vi "生成MES数据串.vi"(7 "测试结果":string, 8 "error in (no error)":errorcluster caption="错误输入（无错误）", 9 "操作状态":T1(ring), 10 "MES配置":T2={"接口地址："="http://192.168.100.120:50000/manufacturing/IntegrationServlet?InterType=XML&message=", "SITE（站点）   "="A155", "PWD（口令）"="LTF", "RESOURCE（资源）"="123456", "OPERATION（工序）"="B03-DZ-ZSCX-01", "USER（用户）"="DZ-ZSCX", "QTY"="LTF", "ACTIVITY"="1", "NC_CODE（NG代码）"="XML", "启用MES"=FALSE}, 11 "ID(SN)":string="A155001") -> (0 "error out":errorcluster caption="错误输出", 2 "Data(OUT)":string="http://192.168.100.120:50000/manufacturing/IntegrationServlet?InterType=XML&message=<PRODUCTION_REQUEST><USER><SITE>A155</SITE><NAME>LTF</NAME><PWD>123456</PWD></USER></PRODUCTION_REQUEST>")   [LabVIEW 2011]
doc: "Power by Antenna~"
panel:
  in  "字符串":string
  out "连接的字符串":string
  out "Data(OUT) 2":string="http://192.168.100.120:50000/manufacturing/IntegrationServlet?InterType=XML&message=<PRODUCTION_REQUEST><USER><SITE>A155</SITE><NAME>LTF</NAME><PWD>123456</PWD></USER></PRODUCTION_REQUEST>"
  # "Name和User有什么\n区别呢？？"
  # "QTY\n默认值为1"
  # "注意中划线和下划线；\n注意大小写；\n注意全角字符和半角字符"
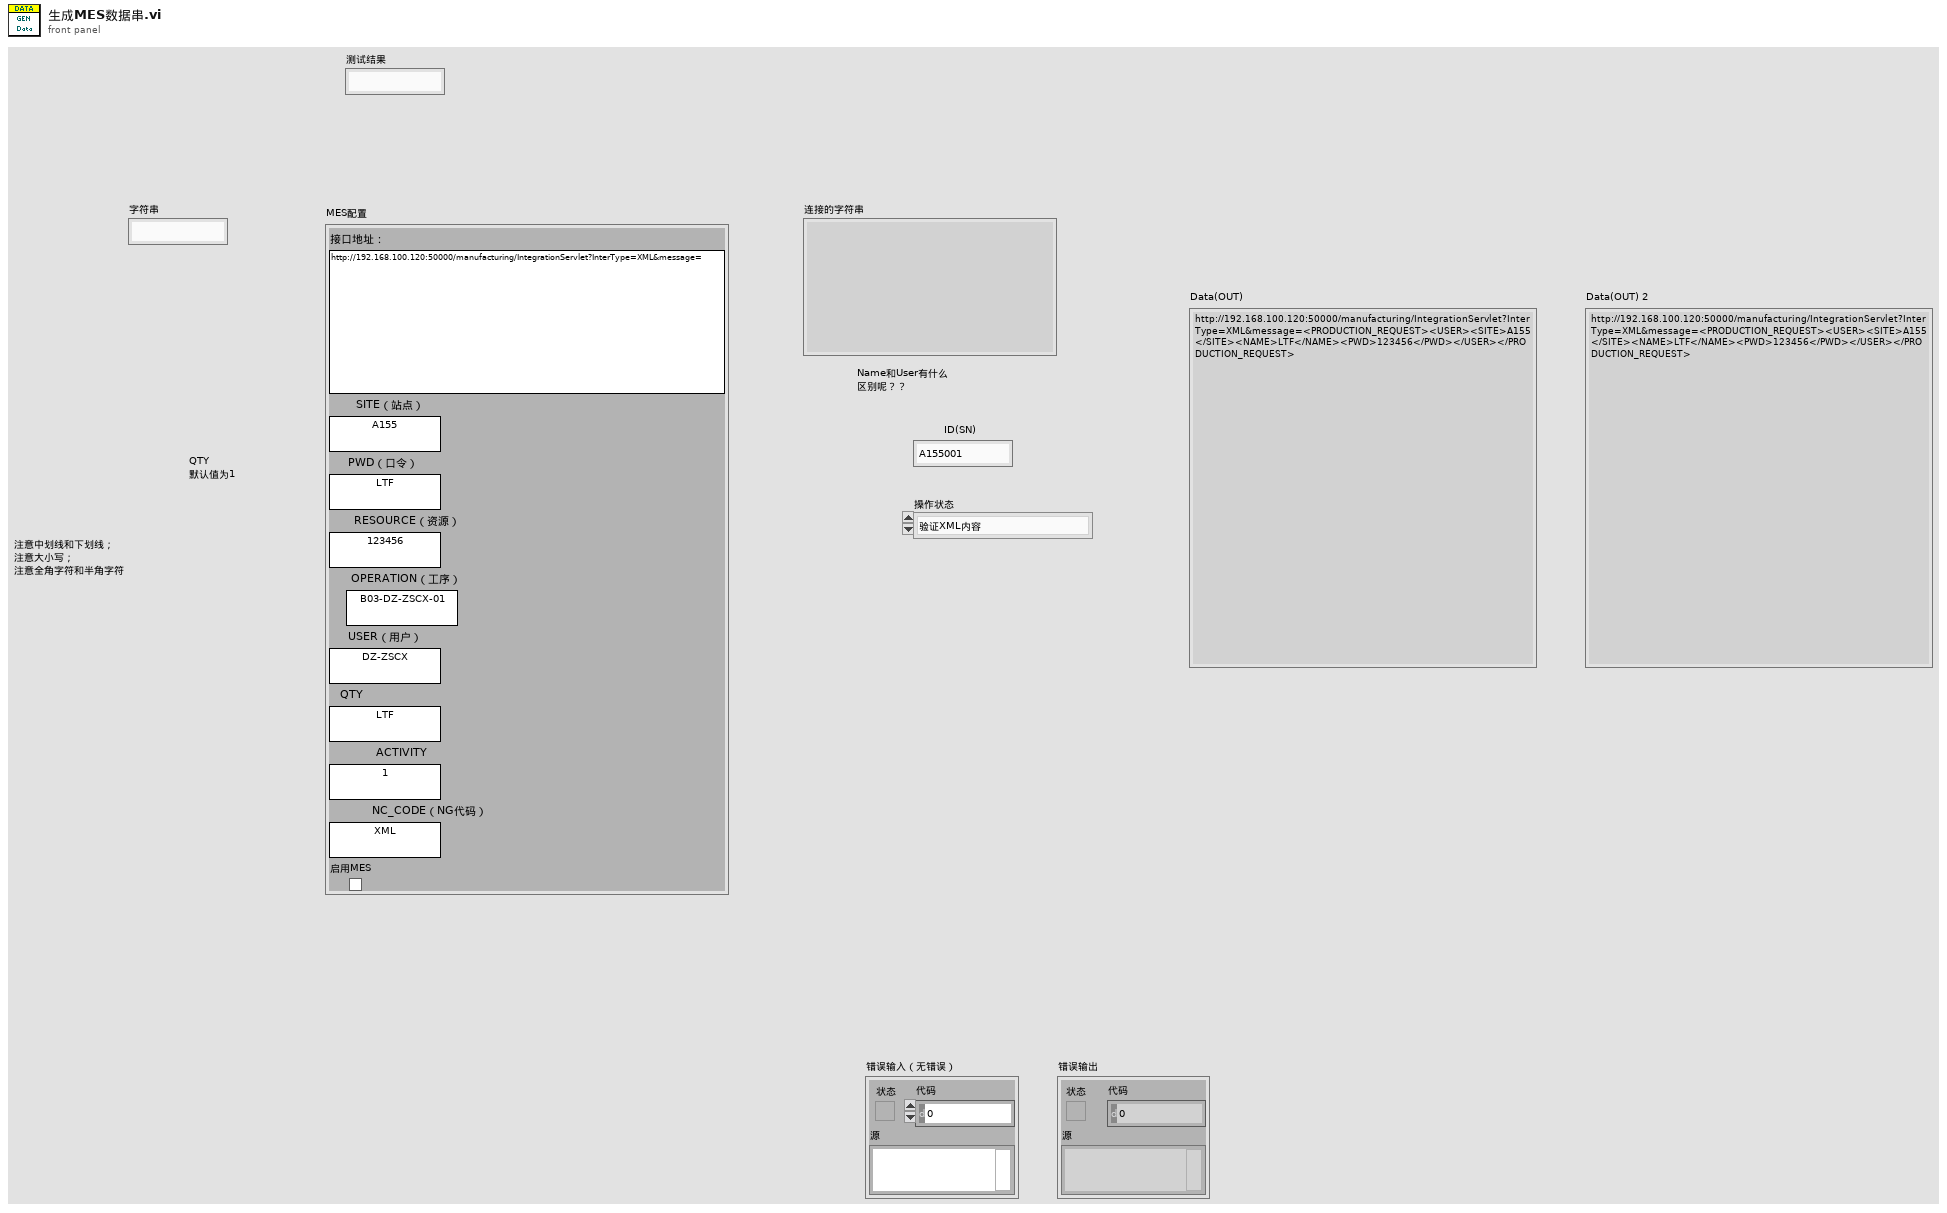
[diagram p1: front panel]
types:
  T1 = enum16{"验证XML内容", "验证条码(Start)", "测试结果合格（PASS）", "测试结果不合格（ERROR）"}
  T2 = typedef "MES设置.ctl" = cluster{"接口地址：":string, "SITE（站点）   ":string, "PWD（口令）":string, "RESOURCE（资源）":string, "OPERATION（工序）":string, "USER（用户）":string, "QTY":string, "ACTIVITY":string, "NC_CODE（NG代码）":string, "启用MES":bool}
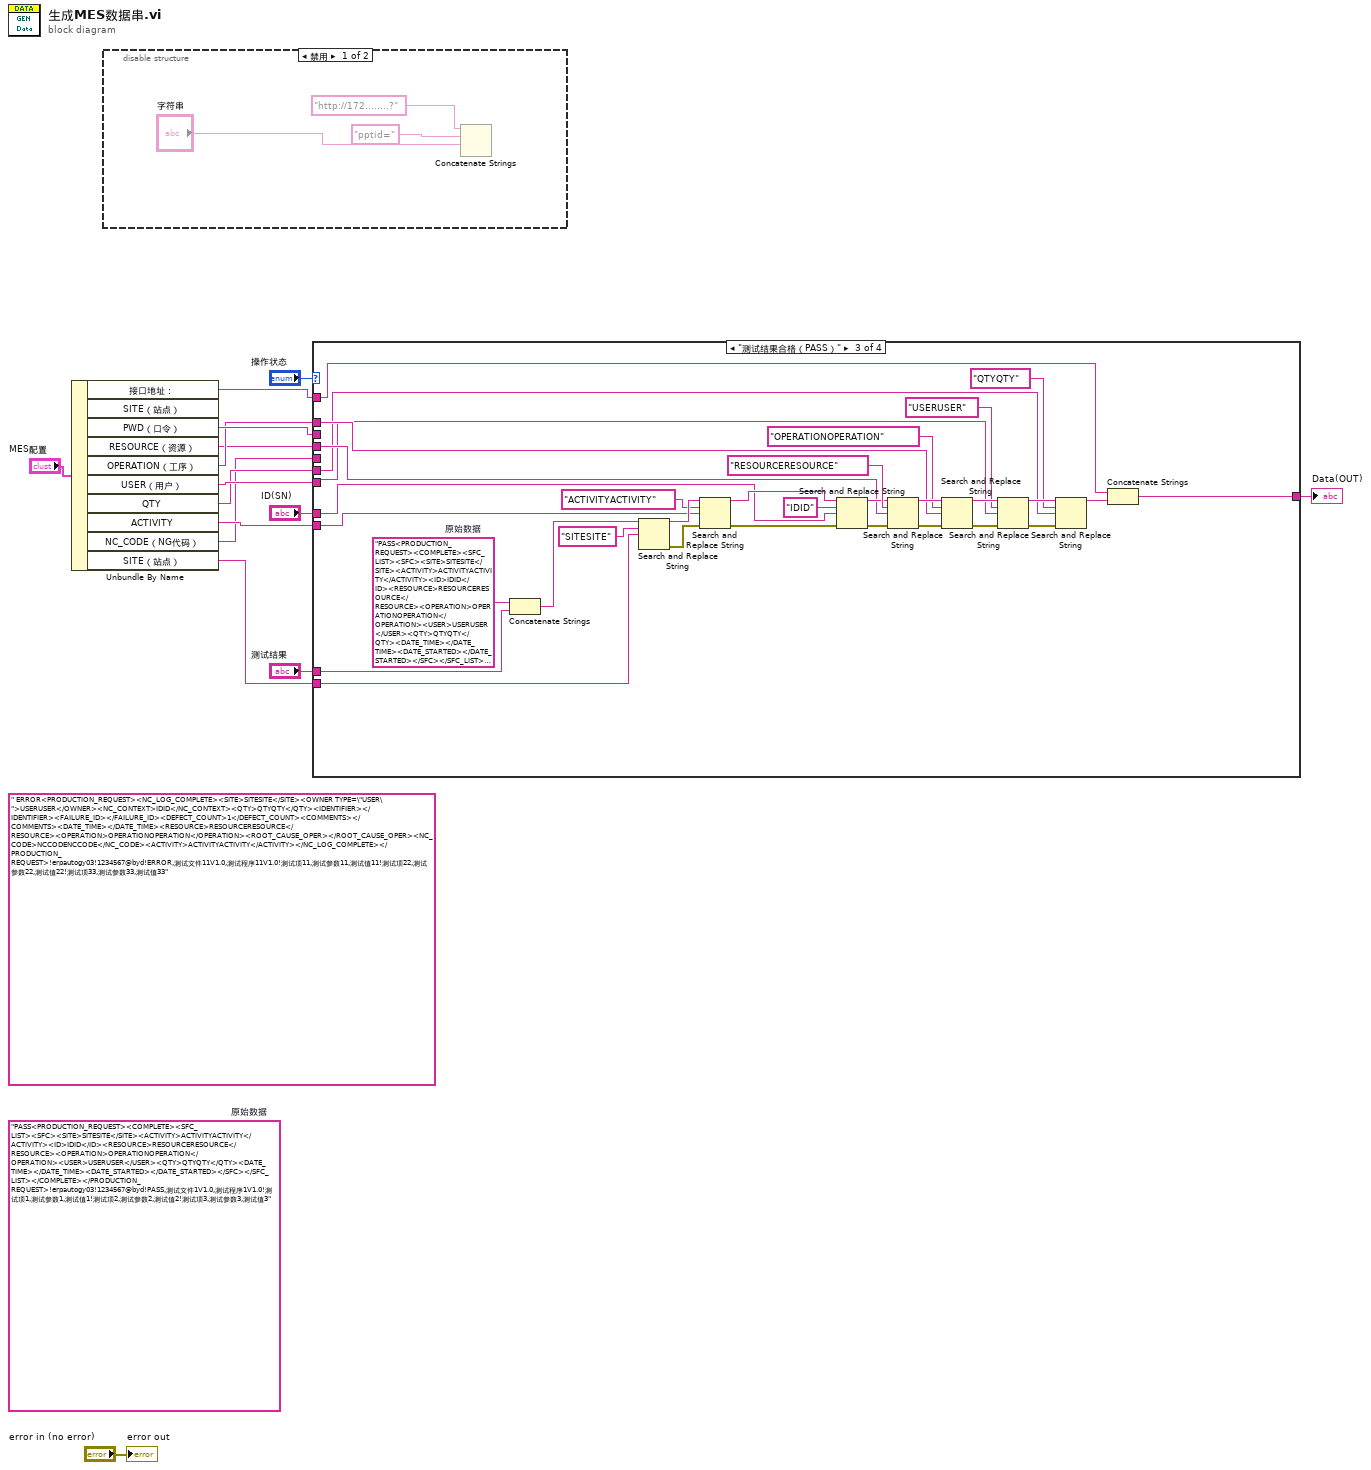
[diagram p0: block diagram]
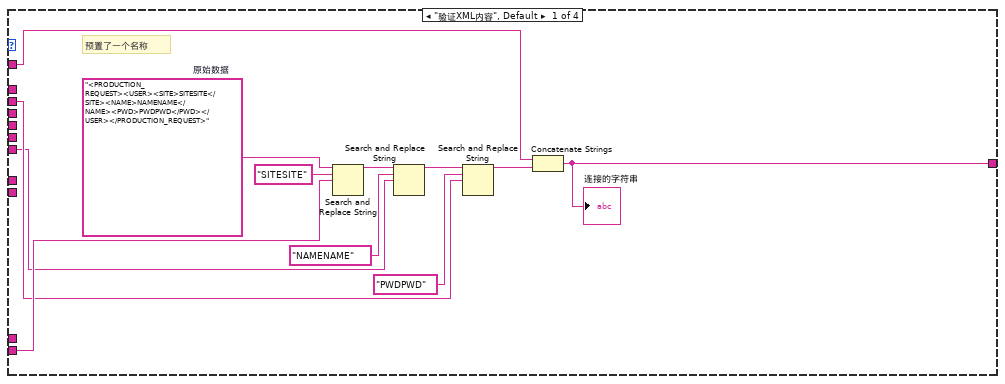
[diagram p3: hidden frame]
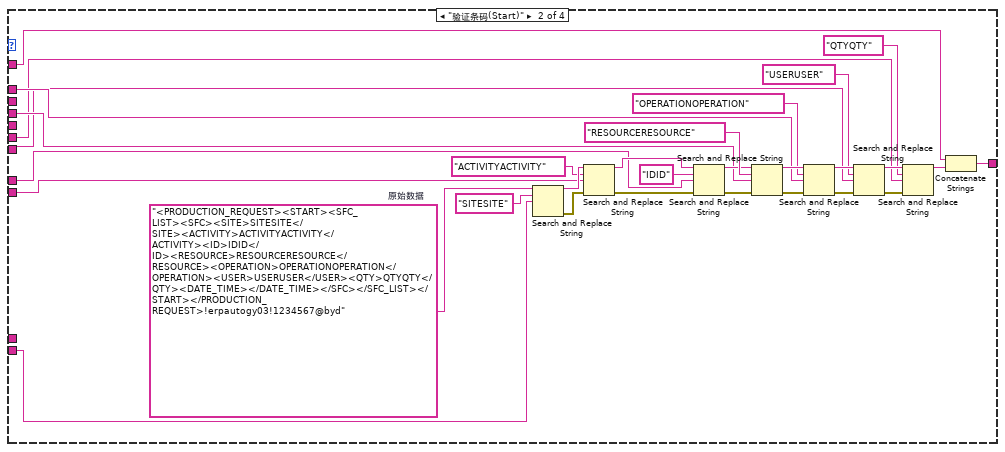
[diagram p4: hidden frame]
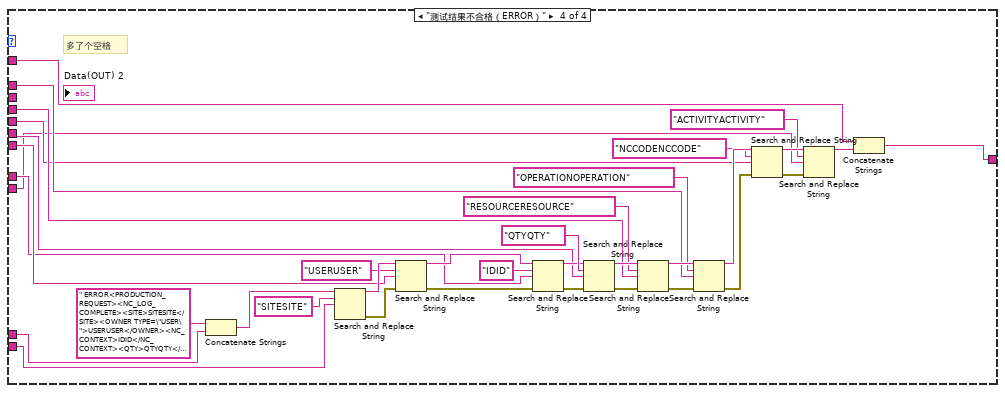
[diagram p5: hidden frame]
diagram:
  (unwired) "PASS<PRODUCTION_REQUEST><COMPLETE><SFC_LIST><SFC><SITE>SITESITE</SITE><ACTIVITY>ACTIVITYACTIVITY</ACTIVITY><ID>IDID</ID><RESOURCE>RESOURCERESOURCE</RESOURCE><OPERATION>OPERATIONOPERATION</OPERATION><USER>USERUSER</USER><QTY>QTYQTY</QTY><DATE_TIME></DATE_TIME><DATE_STARTED></DATE_STARTED></SFC></SFC_LIST></COMPLETE></PRODUCTION_REQUEST>!erpautogy03!1234567@byd!PASS,测试文件1V1.0,测试程序1V1.0!测试项1,测试参数1,测试值1!测试项2,测试参数2,测试值2!测试项3,测试参数3,测试值3"  # 原始数据
  (unwired) " ERROR<PRODUCTION_REQUEST><NC_LOG_COMPLETE><SITE>SITESITE</SITE><OWNER TYPE=\"USER\">USERUSER</OWNER><NC_CONTEXT>IDID</NC_CONTEXT><QTY>QTYQTY</QTY><IDENTIFIER></IDENTIFIER><FAILURE_ID></FAILURE_ID><DEFECT_COUNT>1</DEFECT_COUNT><COMMENTS></COMMENTS><DATE_TIME></DATE_TIME><RESOURCE>RESOURCERESOURCE</RESOURCE><OPERATION>OPERATIONOPERATION</OPERATION><ROOT_CAUSE_OPER></ROOT_CAUSE_OPER><NC_CODE>NCCODENCCODE</NC_CODE><ACTIVITY>ACTIVITYACTIVITY</ACTIVITY></NC_LOG_COMPLETE></PRODUCTION_REQUEST>!erpautogy03!1234567@byd!ERROR,测试文件11V1.0,测试程序11V1.0!测试项11,测试参数11,测试值11!测试项22,测试参数22,测试值22!测试项33,测试参数33,测试值33"
  n1 = Unbundle By Name("MES配置") -> ("接口地址："=w12:string, "PWD（口令）"=w11:string, "RESOURCE（资源）"=w3:string, "OPERATION（工序）"=w10:string, "USER（用户）"=w9:string, "QTY"=w8:string, "ACTIVITY"=w7:string, "NC_CODE（NG代码）"=w6:string, "SITE（站点）"=w1:string)  [unwired: 1 out]
  n2 = disable-structure shown="禁用" {
    frame Disabled {
      n3 = Concatenate Strings("http://172........?", "pptid=" ("字符串"), "字符串") -> ()  [unwired: 1 in, 1 out]
    }
    frame Enabled {
    }
  }
  n4 = case shown="\"测试结果合格（PASS）\"" "操作状态" {
    tunnel: w12 -> [w20 w33 w72 w109]
    tunnel: w1 -> [w24 w52 w70 w107]
    tunnel: w11 -> [w23 _ _ _]
    tunnel: w3 -> [_ w46 w67 w99]
    tunnel: w10 -> [_ w43 w66 w98]
    tunnel: w9 -> [w19 w36 w65 w103]
    tunnel: w8 -> [_ w34 w64 w101]
    tunnel: w7 -> [_ w51 w69 w96]
    tunnel: w6 -> [_ _ _ w97]
    tunnel: [w21 w31 w71 w108] -> w4
    tunnel: "ID(SN)" -> [_ w50 w68 w102]
    tunnel: "测试结果" -> [_ _ w63 w94]
    frame "验证XML内容", Default {
      w30 = "<PRODUCTION_REQUEST><USER><SITE>SITESITE</SITE><NAME>NAMENAME</NAME><PWD>PWDPWD</PWD></USER></PRODUCTION_REQUEST>"  # 原始数据
      # "预置了一个名称"
      n5 = Search and Replace String(input string=w30, search string="SITESITE" ("搜索字符串"), replace string=w24) -> (result string=w27:string)  [unwired: 5 in, 3 out]
      n6 = Search and Replace String(input string=w27, search string="NAMENAME" ("搜索字符串"), replace string=w19) -> (result string=w25:string)  [unwired: 5 in, 3 out]
      n7 = Search and Replace String(input string=w25, search string="PWDPWD" ("搜索字符串"), replace string=w23) -> (result string=w22:string)  [unwired: 5 in, 3 out]
      n8 = Concatenate Strings(w20, w22) -> (w21:string)
      "连接的字符串" <- w21
    }
    frame "验证条码(Start)" {
      w60 = "<PRODUCTION_REQUEST><START><SFC_LIST><SFC><SITE>SITESITE</SITE><ACTIVITY>ACTIVITYACTIVITY</ACTIVITY><ID>IDID</ID><RESOURCE>RESOURCERESOURCE</RESOURCE><OPERATION>OPERATIONOPERATION</OPERATION><USER>USERUSER</USER><QTY>QTYQTY</QTY><DATE_TIME></DATE_TIME></SFC></SFC_LIST></START></PRODUCTION_REQUEST>!erpautogy03!1234567@byd"  # 原始数据
      n9 = Search and Replace String(input string=w60, search string="SITESITE" ("搜索字符串"), replace string=w52) -> (result string=w58:string, error out=w54:errorcluster)  [unwired: 5 in, 2 out]
      n10 = Search and Replace String(input string=w58, search string="ACTIVITYACTIVITY" ("搜索字符串"), replace string=w51, error in=w54) -> (result string=w55:string, error out=w53:errorcluster)  [unwired: 4 in, 2 out]
      n11 = Search and Replace String(input string=w55, search string="IDID" ("搜索字符串"), replace string=w50, error in=w53) -> (result string=w48:string, error out=w47:errorcluster)  [unwired: 4 in, 2 out]
      n12 = Search and Replace String(input string=w48, search string="RESOURCERESOURCE", replace string=w46, error in=w47) -> (result string=w45:string, error out=w40:errorcluster)  [unwired: 4 in, 2 out]
      n13 = Search and Replace String(input string=w45, search string="OPERATIONOPERATION", replace string=w43, error in=w40) -> (result string=w42:string, error out=w41:errorcluster)  [unwired: 4 in, 2 out]
      n14 = Search and Replace String(input string=w42, search string="USERUSER", replace string=w36, error in=w41) -> (result string=w38:string, error out=w39:errorcluster)  [unwired: 4 in, 2 out]
      n15 = Search and Replace String(input string=w38, search string="QTYQTY", replace string=w34, error in=w39) -> (result string=w32:string)  [unwired: 4 in, 3 out]
      n16 = Concatenate Strings(w33, w32) -> (w31:string)
    }
    frame "测试结果合格（PASS）" {
      w62 = "PASS<PRODUCTION_REQUEST><COMPLETE><SFC_LIST><SFC><SITE>SITESITE</SITE><ACTIVITY>ACTIVITYACTIVITY</ACTIVITY><ID>IDID</ID><RESOURCE>RESOURCERESOURCE</RESOURCE><OPERATION>OPERATIONOPERATION</OPERATION><USER>USERUSER</USER><QTY>QTYQTY</QTY><DATE_TIME></DATE_TIME><DATE_STARTED></DATE_STARTED></SFC></SFC_LIST></COMPLETE></PRODUCTION_REQUEST>!erpautogy03!1234567@byd!PASS,测试文件1V1.0,测试程序1V1.0!"  # 原始数据
      n17 = Concatenate Strings(w62, w63) -> (w61:string)
      n18 = Search and Replace String(input string=w61, search string="SITESITE" ("搜索字符串"), replace string=w70) -> (result string=w91:string, error out=w89:errorcluster)  [unwired: 5 in, 2 out]
      n19 = Search and Replace String(input string=w91, search string="ACTIVITYACTIVITY" ("搜索字符串"), replace string=w69, error in=w89) -> (result string=w87:string, error out=w88:errorcluster)  [unwired: 4 in, 2 out]
      n20 = Search and Replace String(input string=w87, search string="IDID" ("搜索字符串"), replace string=w68, error in=w88) -> (result string=w84:string, error out=w83:errorcluster)  [unwired: 4 in, 2 out]
      n21 = Search and Replace String(input string=w84, search string="RESOURCERESOURCE", replace string=w67, error in=w83) -> (result string=w82:string, error out=w81:errorcluster)  [unwired: 4 in, 2 out]
      n22 = Search and Replace String(input string=w82, search string="OPERATIONOPERATION", replace string=w66, error in=w81) -> (result string=w79:string, error out=w78:errorcluster)  [unwired: 4 in, 2 out]
      n23 = Search and Replace String(input string=w79, search string="USERUSER", replace string=w65, error in=w78) -> (result string=w76:string, error out=w75:errorcluster)  [unwired: 4 in, 2 out]
      n24 = Search and Replace String(input string=w76, search string="QTYQTY", replace string=w64, error in=w75) -> (result string=w73:string)  [unwired: 4 in, 3 out]
      n25 = Concatenate Strings(w72, w73) -> (w71:string)
    }
    frame "测试结果不合格（ERROR）" {
      # "多了个空格"
      n26 = Concatenate Strings(" ERROR<PRODUCTION_REQUEST><NC_LOG_COMPLETE><SITE>SITESITE</SITE><OWNER TYPE=\"USER\">USERUSER</OWNER><NC_CONTEXT>IDID</NC_CONTEXT><QTY>QTYQTY</QTY><IDENTIFIER></IDENTIFIER><FAILURE_ID></FAILURE_ID><DEFECT_COUNT>1</DEFECT_COUNT><COMMENTS></COMMENTS><DATE_TIME></DATE_TIME><RESOURCE>RESOURCERESOURCE</RESOURCE><OPERATION>OPERATIONOPERATION</OPERATION><ROOT_CAUSE_OPER></ROOT_CAUSE_OPER><NC_CODE>NCCODENCCODE</NC_CODE><ACTIVITY>ACTIVITYACTIVITY</ACTIVITY></NC_LOG_COMPLETE></PRODUCTION_REQUEST>!erpautogy03!1234567@byd!ERROR,测试文件11V1.0,测试程序11V1.0!", w94) -> (w93:string)
      n27 = Search and Replace String(input string=w93, search string="SITESITE" ("搜索字符串"), replace string=w107) -> (result string=w127:string, error out=w125:errorcluster)  [unwired: 5 in, 2 out]
      n28 = Search and Replace String(input string=w127, search string="USERUSER" ("搜索字符串"), replace string=w103, error in=w125) -> (result string=w123:string, error out=w124:errorcluster)  [unwired: 4 in, 2 out]
      n29 = Search and Replace String(input string=w123, search string="IDID" ("搜索字符串"), replace string=w102, error in=w124) -> (result string=w120:string, error out=w119:errorcluster)  [unwired: 4 in, 2 out]
      n30 = Search and Replace String(input string=w120, search string="QTYQTY", replace string=w101, error in=w119) -> (result string=w118:string, error out=w117:errorcluster)  [unwired: 4 in, 2 out]
      n31 = Search and Replace String(input string=w118, search string="RESOURCERESOURCE", replace string=w99, error in=w117) -> (result string=w115:string, error out=w114:errorcluster)  [unwired: 4 in, 2 out]
      n32 = Search and Replace String(input string=w115, search string="OPERATIONOPERATION", replace string=w98, error in=w114) -> (result string=w112:string, error out=w111:errorcluster)  [unwired: 4 in, 2 out]
      n33 = Search and Replace String(input string=w112, search string="NCCODENCCODE", replace string=w97, error in=w111) -> (result string=w106:string, error out=w105:errorcluster)  [unwired: 4 in, 2 out]
      n34 = Search and Replace String(input string=w106, search string="ACTIVITYACTIVITY" ("搜索字符串"), replace string=w96, error in=w105) -> (result string=w104:string)  [unwired: 4 in, 3 out]
      n35 = Concatenate Strings(w109, w104) -> (w108:string)
    }
  }
  "Data(OUT)" <- w4
  "error out" <- "error in (no error)"
